vi "DataArray_Formatter.vi"(0 "PartitionArray":string[](array[string]), 1 "Temps":dbl[][](graph), 2 "FrozenFraction":dbl[](array[numeric]), 3 "FreezeTemps":dbl[](array[numeric]), 4 "Offsets":dbl[](array[numeric]), 5 "Offset Applied?":bool, 6 "input cluster":T1={"Core"={"Current VI Reference"=refnum, "Close Panel on Exit?"=FALSE}, "Image Out"=refnum, "State"=0, "Points"={"Top Left"={"X"=0.0, "Y"=0.0}, "Top Right"={"X"=0.0, "Y"=0.0}, "Bottom Left"={"X"=0.0, "Y"=0.0}, "Bottom Right"={"X"=0.0, "Y"=0.0}, "x space 2"=0.0, "y space 2"=0.0, "x_space"=0.0, "y_space"=0.0, "Pixels"=[], "Fixpoint"={"X"=0.0, "Y"=0.0}}, "img_array"=[], "Temps"=[], "Temps_Array"=[], "Scan Area"=0.0, "Fixpoint Area"=0.0, "Config"={"Freezing"={"Cutoff"=2.0}}, "PCR Size"=0} {"Points"."Bottom Right"."Y" format="%.2f"; "Points"."Bottom Right"."X" format="%.2f"; "Points"."Top Left"."Y" format="%.2f"; "Points"."Top Left"."X" format="%.2f"; "Points"."Top Right"."Y" format="%.2f"; "Points"."Top Right"."X" format="%.2f"; "Points"."Bottom Left"."Y" format="%.2f"; "Points"."Bottom Left"."X" format="%.2f"; "Points"."Fixpoint"."Y" format="%.2f"; "Points"."Fixpoint"."X" format="%.2f"}, 9 "MeltTemps":dbl[](array[numeric])) -> (14 "Data Array":string[][](array[string]))   [LabVIEW 2020]
uses:
  DataCluster_TCAL.ctl
  <vilib>/vision/Image Controls.llb/IMAQ Image.ctl
  TCE_Config.ctl
panel:
  out "appended array":string[][](array[string])
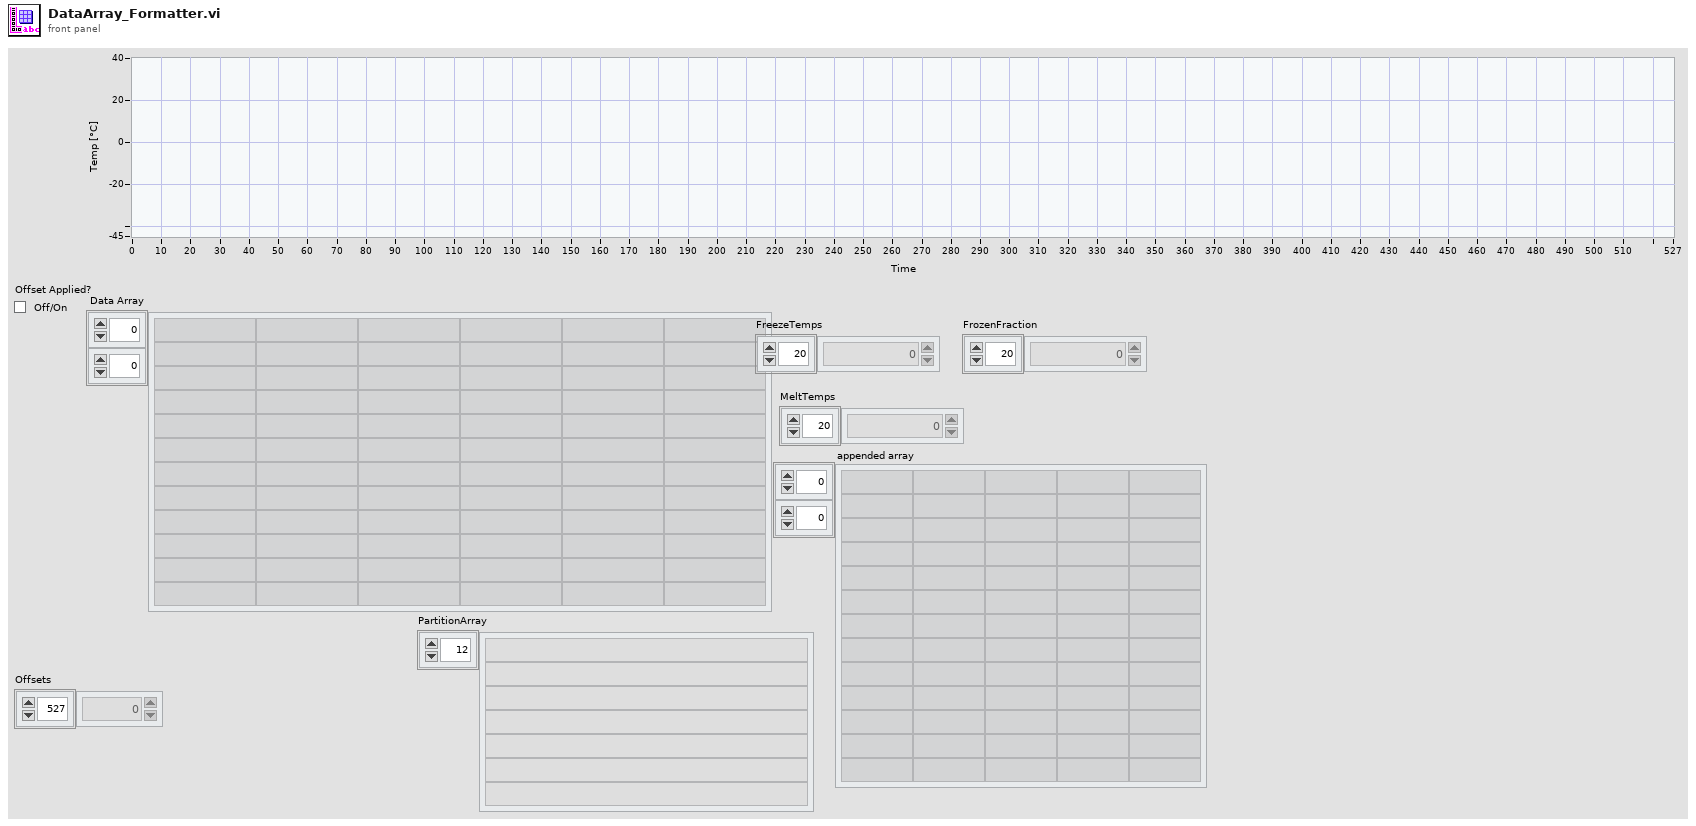
[diagram p1: front panel]
types:
  T1 = typedef "DataCluster_TCAL.ctl" = cluster{"Core":cluster{"Current VI Reference":refnum<vi>, "Close Panel on Exit?":bool}, "Image Out":T2, "State":i32, "Points":cluster{"Top Left":T3, "Top Right":T3, "Bottom Left":T3, "Bottom Right":T3, "x space 2":dbl, "y space 2":sgl, "x_space":sgl, "y_space":sgl, "Pixels":cluster{"X":i32, "Y":i32}[][], "Fixpoint":T3}, "img_array":T2[], "Temps":dbl[], "Temps_Array":dbl[][], "Scan Area":dbl, "Fixpoint Area":dbl, "Config":T4, "PCR Size":u16}
  T2 = typedef "IMAQ Image.ctl" = refnum<image>
  T3 = typedef "IMAQ Point" = cluster{"X":sgl, "Y":sgl}
  T4 = typedef "TCE_Config.ctl" = cluster{"Freezing":cluster{"Cutoff":dbl}}
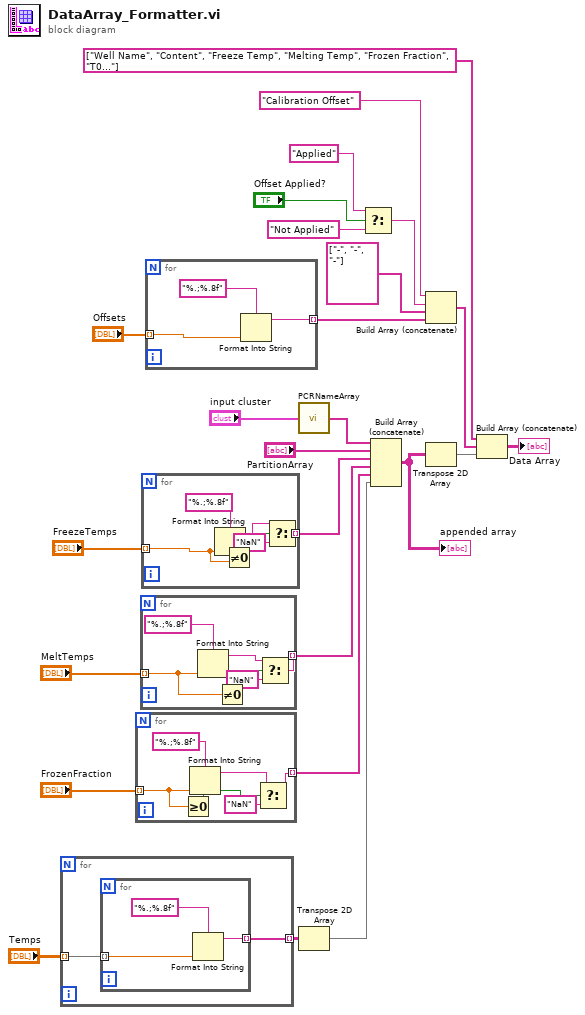
[diagram p0: block diagram]
diagram:
  n1 = for {
    tunnel: "Temps" -> [w27] mode=indexing
    tunnel: [w26] -> w18 mode=indexing
    n2 = for {
      tunnel: w27 -> [w30] mode=indexing
      tunnel: [w29] -> w26 mode=indexing
      n3 = Format Into String(format string="%.;%.8f", w30) -> (resulting string=w29:string)  [unwired: 2 in, 1 out]
    }
  }
  n4 = for {
    tunnel: "FrozenFraction" -> [w33] mode=indexing
    tunnel: [w34] -> w1 mode=indexing
    n5 = Greater Or Equal To 0?(x=w33) -> (x >= 0?=w32:bool)
    n6 = Format Into String(format string="%.;%.8f", w33) -> (resulting string=w35:string)  [unwired: 2 in, 1 out]
    n7 = Select(t=w35, s=w32, f="NaN") -> (s? t:f=w34:string)
  }
  n8 = for {
    tunnel: "MeltTemps" -> [w37] mode=indexing
    tunnel: [w40] -> w6 mode=indexing
    n9 = Format Into String(format string="%.;%.8f", w37) -> (resulting string=w39:string)  [unwired: 2 in, 1 out]
    n10 = Not Equal To 0?(x=w37) -> (x != 0?=w38:bool)
    n11 = Select(t=w39, s=w38, f="NaN") -> (s? t:f=w40:string)
  }
  n12 = for {
    tunnel: "FreezeTemps" -> [w44] mode=indexing
    tunnel: [w47] -> w20 mode=indexing
    n13 = Format Into String(format string="%.;%.8f", w44) -> (resulting string=w46:string)  [unwired: 2 in, 1 out]
    n14 = Not Equal To 0?(x=w44) -> (x != 0?=w45:bool)
    n15 = Select(t=w46, s=w45, f="NaN") -> (s? t:f=w47:string)
  }
  n16 = for {
    tunnel: "Offsets" -> [w51] mode=indexing
    tunnel: [w50] -> w5 mode=indexing
    n17 = Format Into String(format string="%.;%.8f", w51) -> (resulting string=w50:string)  [unwired: 2 in, 1 out]
  }
  n18 = call "PCRNameArray.vi"("input cluster"="input cluster") -> ("WellArray"=w25:string[])
  n19 = Transpose 2D Array(2D array=w18) -> (transposed array=w2:string[][])
  n20 = Select(t="Applied", s="Offset Applied?", f="Not Applied") -> (s? t:f=w8:string)
  n21 = Build Array (concatenate)(w25, "PartitionArray", w20, w6, w1, w2) -> (w22:string[][])
  "appended array" <- w22
  n22 = Build Array (concatenate)("Calibration Offset" ("element"), w8, string[] ["-", "-", "-"] ("array"), w5) -> (w13:string[])
  n23 = Transpose 2D Array(2D array=w22) -> (transposed array=w21:string[][])
  n24 = Build Array (concatenate)(string[] ["Well Name", "Content", "Freeze Temp", "Melting Temp", "Frozen Fraction", "T0..."], w13, w21) -> (→"Data Array":string[][])
